vi "Is Source.vi"(8 "error in (no error)":errorcluster, 11 "terminal in":refnum<vi>) -> (0 "error out":errorcluster, 2 "is source":bool, 3 "terminal out":refnum<vi>)   [LabVIEW 2017]
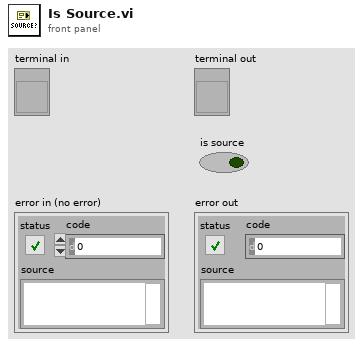
[diagram p1: front panel]
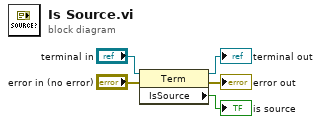
[diagram p0: block diagram]
diagram:
  n1 = property class="Term"(reference="terminal in", error in="error in (no error)") -> (reference out=→"terminal out":refnum<vi>, error out=→"error out":errorcluster, "IsSource"=→"is source":bool)
